vi "Measurement Logic.vi"() -> ()   [LabVIEW 2021, in "ImageRendering.lvlib"]
uses:
  ImageRendering.lvlib
  Measurement Configuration.ctl
  Measurement Results.ctl
  <vilib>/MeasurementLink/MeasurementLink Measurement Server/Measure Call Context/Measure Call Context.lvclass
  <vilib>/vision/driver/IMAQdx.llb/IMAQdx Camera Control Mode.ctl
  <vilib>/vision/driver/IMAQdx.llb/IMAQdx Acquisition Mode.ctl
  <vilib>/MeasurementLink/MeasurementLink Measurement Server/Measure Call Context/Accessor/Is Canceled.vi
  <vilib>/vision/driver/NI_Vision_Acquisition_Software.lvlib
panel:
  out "Acquired Frames per Second":dbl
  out "measure call context out":refnum<class "Measure Call Context.lvclass">
  in  "measure call context in":refnum<class "Measure Call Context.lvclass">
  out "measurement results":T1={"Image Data"="Empty", "Image Resolution"=[], "Image Pixels (U32)"=[], "Last Buffer Number"=0}
  in  "measurement configuration":T2={"Camera name"="D:\\Avi\\_PRK5307.jpg", "Image Converison Type"=""}
  out "error out":errorcluster
  in  "error in":errorcluster
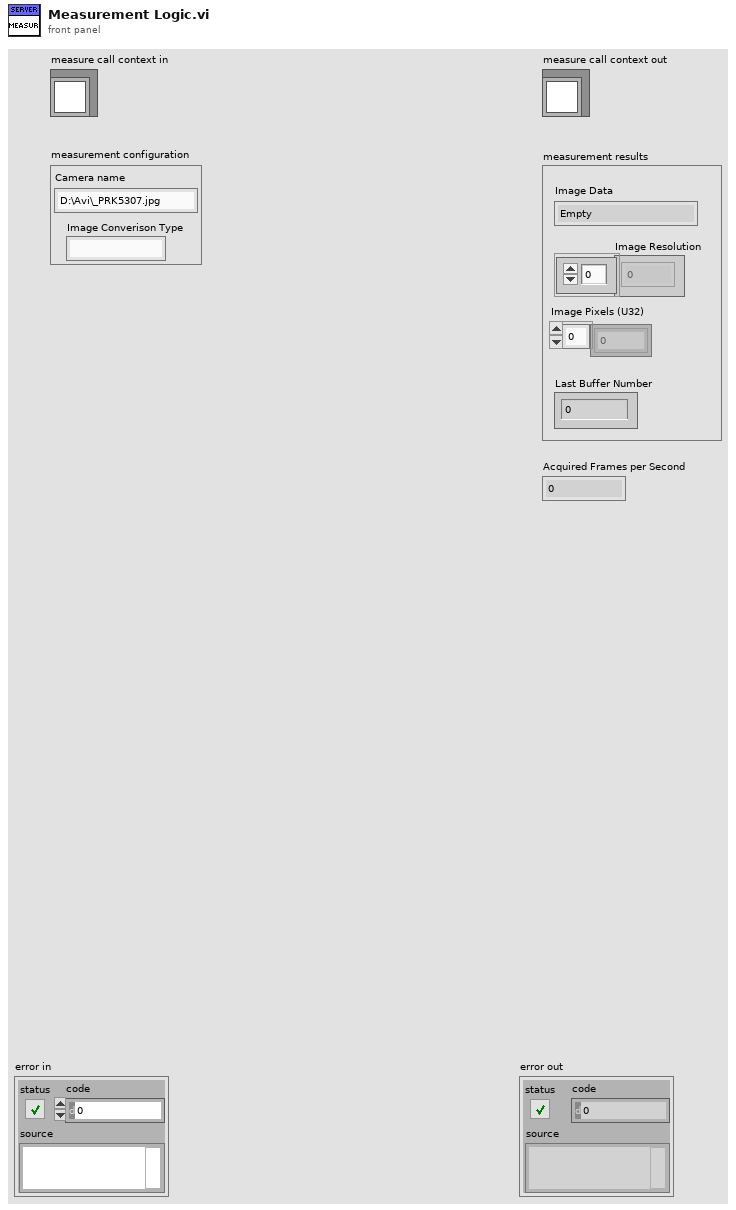
[diagram p1: front panel]
types:
  T1 = typedef "ImageRendering.lvlib/Measurement Results.ctl" = cluster{"Image Data":string, "Image Resolution":i32[], "Image Pixels (U32)":u32[], "Last Buffer Number":u32}
  T2 = typedef "ImageRendering.lvlib/Measurement Configuration.ctl" = cluster{"Camera name":string, "Image Converison Type":string}
  T3 = typedef "NI_Vision_Acquisition_Software.lvlib/IMAQdx Acquisition Mode.ctl" = enum32{"One Shot", "Continuous"}
  T4 = typedef "NI_Vision_Acquisition_Software.lvlib/IMAQdx Camera Control Mode.ctl" = enum32{"Controller", "Listener"}
  T5 = typedef "IMAQdx.ctl" = refnum<k21>
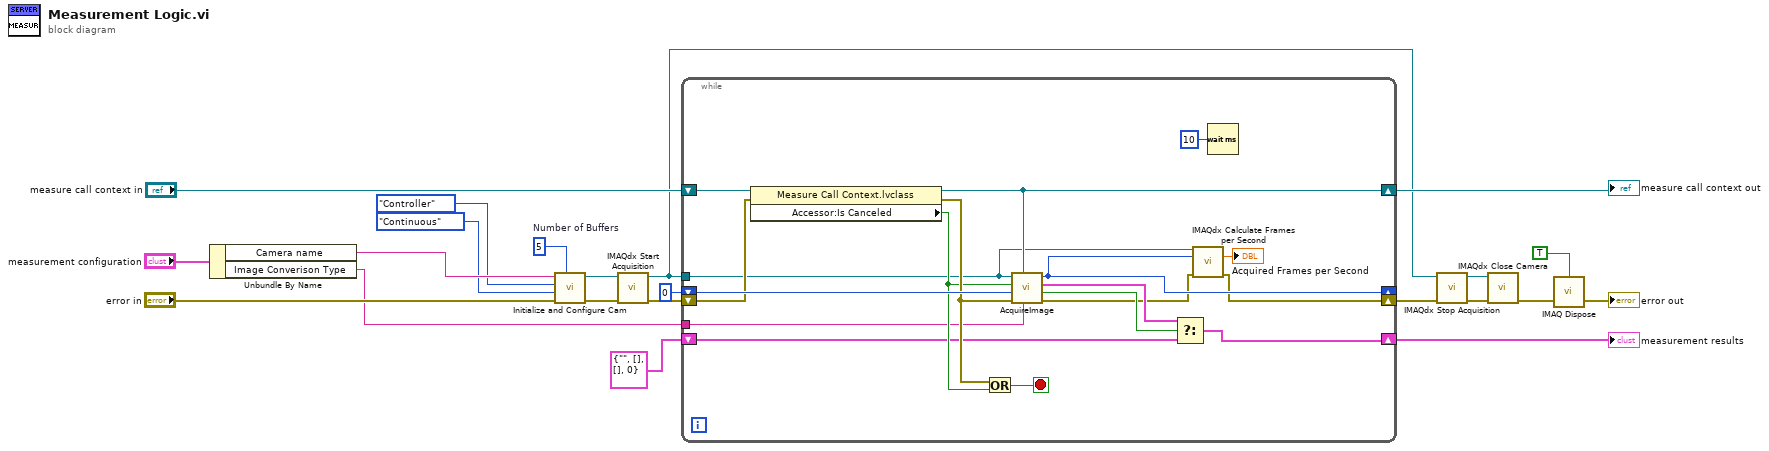
[diagram p0: block diagram]
diagram:
  w16 = u32 5  # Number of Buffers
  n1 = Unbundle By Name("measurement configuration") -> ("Camera name"=w21:string, "Image Converison Type"=w10:string)
  n2 = call "Initialize and Configure Cam.vi"("Number of Buffers"=w16, "error in"="error in", "Continuous?"=IMAQdx_Acquisition_Mode."Continuous", "Camera Control Mode"=IMAQdx_Camera_Control_Mode."Controller", "Camera name"=w21) -> ("error out"=w20:errorcluster, "camera session out"=w19:T5)  [unwired: 5 in]
  n3 = call <vilib>:"IMAQdx Start Acquisition.vi"("error in"=w20, "Session In"=w19) -> ("error out"=w12:errorcluster, "Session Out"=w6:T5)  [unwired: 8 in]
  n4 = while {
    shift-right: [w33] -> w13
    shift-left: "measure call context in" -> [w40]
    tunnel: w6 -> [w27]
    shift-right: [w26] -> _
    shift-left: u32 0 ("Buffer Number Out") -> [w39]
    tunnel: w10 -> [w34]
    shift-right: [w29] -> w8
    shift-left: T1 {"Image Data"="", "Image Resolution"=[], "Image Pixels (U32)"=[], "Last Buffer Number"=0} ("Measurement Results") -> [w30]
    shift-right: [w24] -> w7
    shift-left: w12 -> [w38]
    stop <- w36 stop-if-true
    n5 = property class="Measure Call Context.lvclass"(reference=w40, error in=w38) -> (reference out=w33:refnum<class "Measure Call Context.lvclass">, error out=w37:errorcluster, "Accessor:Is Canceled"=w35:bool)
    n6 = Or(x=w37, y=w35) -> (x .or. y?=w36:bool)
    n7 = call "AcquireImage.vi"("Image Conversion"=w34, "measure call context in"=w33, "error in (no error)"=w37, "Buffer Number Out in"=w39, "Accessor:Is Canceled"=w35, "Refnum in"=w27) -> ("error out"=w25:errorcluster, "Valid Result"=w32:bool, "Measurement Results"=w31:T1, "Buffer Number Out out"=w26:u32)  [unwired: 2 in]
    n8 = Select(t=w31, s=w32, f=w30) -> (s? t:f=w29:T1)
    n9 = call <vilib>:"IMAQdx Calculate Frames per Second.vi"("Session In"=w27, "Buffer Number"=w26, "error in (no error)"=w25) -> ("Acquired Frames per Second"=→"Acquired Frames per Second":dbl, "error out"=w24:errorcluster)  [unwired: 6 in, 5 out]
    n10 = Wait (ms)(milliseconds to wait=u32 10) -> ()  [unwired: 1 out]
  }
  "measurement results" <- w8
  "measure call context out" <- w13
  n11 = call <vilib>:"IMAQdx Stop Acquisition.vi"("error in"=w7, "Session In"=w6) -> ("error out"=w4:errorcluster, "Session Out"=w5:T5)  [unwired: 8 in]
  n12 = call <vilib>:"IMAQdx Close Camera.vi"("error in"=w4, "Session In"=w5) -> ("error out"=w3:errorcluster)  [unwired: 9 in]
  n13 = call "IMAQ Dispose"("All Images? (No)"=TRUE, "error in (no error)"=w3) -> ("error out"=→"error out":errorcluster)  [unwired: 4 in]
